vi "Read Init Motor Data.vi"(8 "error in (no error)":errorcluster, 11 "SGDV_Ctrl_Class in":refnum<class "SGDV Motor.lvclass">) -> (0 "error out":errorcluster, 1 "Init Motor Data":T1, 2 "Get Serial Data?":bool, 3 "SGDV_Ctrl_Class out":refnum<class "SGDV Motor.lvclass">)   [LabVIEW 2013, in "SGDV_Ctrl_v13_lib.lvlib" / "SGDV Motor.lvclass"]
uses:
  SGDV Motor.lvclass
  Controls and General VIs/Init Motor Data.ctl
  SGDV Motor.lvclass/SGDV Motor.ctl
  Controls and General VIs/Delta FPGA Refnum.ctl
  <vilib>/myRIO/Common/Instrument Driver Framework/myRIO v1.0/Encoder/typedefs/Encoder Signal Mode.ctl
  <vilib>/rvi/interface/common/niFpgaWaitOnOcc.vi
  <vilib>/myRIO/Instrument Drivers/Onboard IO/Encoder/vis/Open.vi
  <vilib>/myRIO/Common/Instrument Driver Framework/myRIO v1.0/Encoder/vis/myRIO v1.1 Open Encoder.vi
  <vilib>/myRIO/Common/Instrument Driver Framework/myRIO v1.0/Encoder/vis/myRIO v1.0 Close Encoder.vi
  <vilib>/myRIO/Common/Instrument Driver Framework/Utilities/vis/Validate Channels.vi
  <vilib>/myRIO/Common/Instrument Driver Framework/myRIO v1.0/Encoder/vis/myRIO v1.0 Reserve Encoder.vi
  <vilib>/myRIO/Common/Instrument Driver Framework/myRIO v1.0/Encoder/vis/myRIO v1.0 Unreserve Encoder.vi
  <vilib>/myRIO/Common/Instrument Driver Framework/myRIO v1.0/Encoder/vis/myRIO v1.0 Build MUX Configuration Encoder.vi
  <vilib>/myRIO/Common/Instrument Driver Framework/myRIO v1.0/Resource Manager/vis/myRIO v1.0 Reserve Channel List.vi
  <vilib>/myRIO/Common/Instrument Driver Framework/myRIO v1.0/Resource Manager/vis/myRIO v1.0 Unreserve Channel List.vi
  <vilib>/myRIO/Common/Instrument Driver Framework/myRIO v1.0/Resource Manager/vis/myRIO v1.0 Create Configuration List.vi
  <vilib>/myRIO/Common/Instrument Driver Framework/myRIO v1.0/Resource Manager/vis/myRIO v1.0 Reserve Channel.vi
  <vilib>/myRIO/Common/Instrument Driver Framework/myRIO v1.0/Resource Manager/vis/myRIO v1.0 Unreserve Channel.vi
  <vilib>/myRIO/Common/Instrument Driver Framework/myRIO v1.0/Resource Manager/vis/myRIO v1.0 Build Mutex Name.vi
  <vilib>/myRIO/Common/Instrument Driver Framework/myRIO v1.0/Encoder/vis/myRIO v1.0 Configure Encoder.vi
  <vilib>/myRIO/Common/Instrument Driver Framework/myRIO v1.0/myRIO v1.1 Open.vi
  <vilib>/Utility/VariantDataType/GetNumericInfo.vi
  <vilib>/Utility/error.llb/Error Cluster From Error Code.vi
  <vilib>/myRIO/Common/Instrument Driver Framework/Utilities/vis/IO Manager.vi
  <vilib>/myRIO/Common/Instrument Driver Framework/Utilities/vis/Configuration Manager.vi
  <vilib>/myRIO/Common/Instrument Driver Framework/myRIO v1.0/Resource Manager/vis/myRIO v1.0 Configure IO.vi
  <vilib>/myRIO/Common/Instrument Driver Framework/myRIO v1.0/myRIO v1.0 Close.vi
  <vilib>/myRIO/Common/Instrument Driver Framework/myRIO v1.0/Encoder/vis/myRIO v1.0 Shutdown Encoder.vi
  <vilib>/myRIO/Common/Instrument Driver Framework/myRIO v1.0/Encoder/vis/myRIO v1.0 Read Encoder.vi
  <vilib>/rvi/errors/niLvFpgaAdjustHostInterfaceError.vi
  <vilib>/rvi/interface/nirviReadWriteControl/nirviReadWriteControl.xnode
  <vilib>/rvi/interface/nirviMethod/nirviMethod.xnode
  SGDV_Ctrl_v13_lib.lvlib
  NiFpgaLv.dll
  <vilib>/rvi/interface/Simulation/niFpgaSimulationCallBeginRW.vi
  <vilib>/myRIO/Instrument Drivers/Onboard IO/Encoder/Encoder.lvlib
  <vilib>/FPGAPlugInAG/Dynamic/niLvFpga_ReadFifo_Dynamic.vi
  <vilib>/rvi/errors/niLvFpgaMergeErrorWithErrorCode.vi
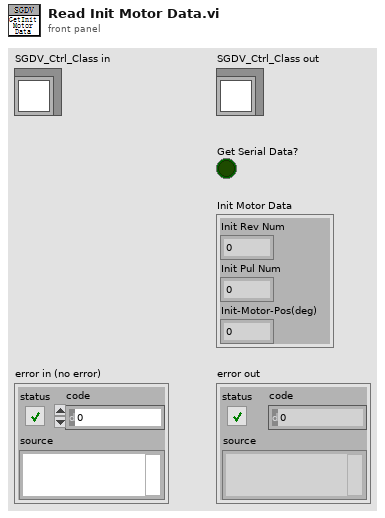
[diagram p1: front panel]
types:
  T1 = typedef "SGDV_Ctrl_v13_lib.lvlib/Init Motor Data.ctl" = cluster{"Init Rev Num":i32, "Init Pul Num":i32, "Init-Motor-Pos(deg)":dbl}
  T2 = typedef "Generic FPGA Reference.ctl" = refnum<k20>
  T3 = typedef "SGDV_Ctrl_v13_lib.lvlib/Delta FPGA Refnum.ctl" = refnum<k20>
  T4 = typedef "Encoder Signal Mode.ctl" = enum16{"Quadrature Phase Signal", "Step and Direction Signal"}
  T5 = typedef "Encoder.lvlib/Encoder Reference.ctl" = cluster{"myRIO Reference":T6, "Encoder Channels Enum":T9}
  T6 = typedef "myRIO Generic Hardware Reference.ctl" = cluster{"myRIO Model":T7, "myRIO Hardware Reference":T8}
  T7 = typedef "Hardware Version Enum.ctl" = enum16{"Unknown", "myRIO-1900", "myRIO-1950"}
  T8 = typedef "myRIO v1.0 Reference.ctl" = cluster{"Generic FPGA Reference":T2, "Allow multiple opens":bool}
  T9 = typedef "Encoder Channels Enum.ctl" = enum16{"Not Connected", "C/ENC0", "C/ENC1", "A/ENC", "B/ENC"}
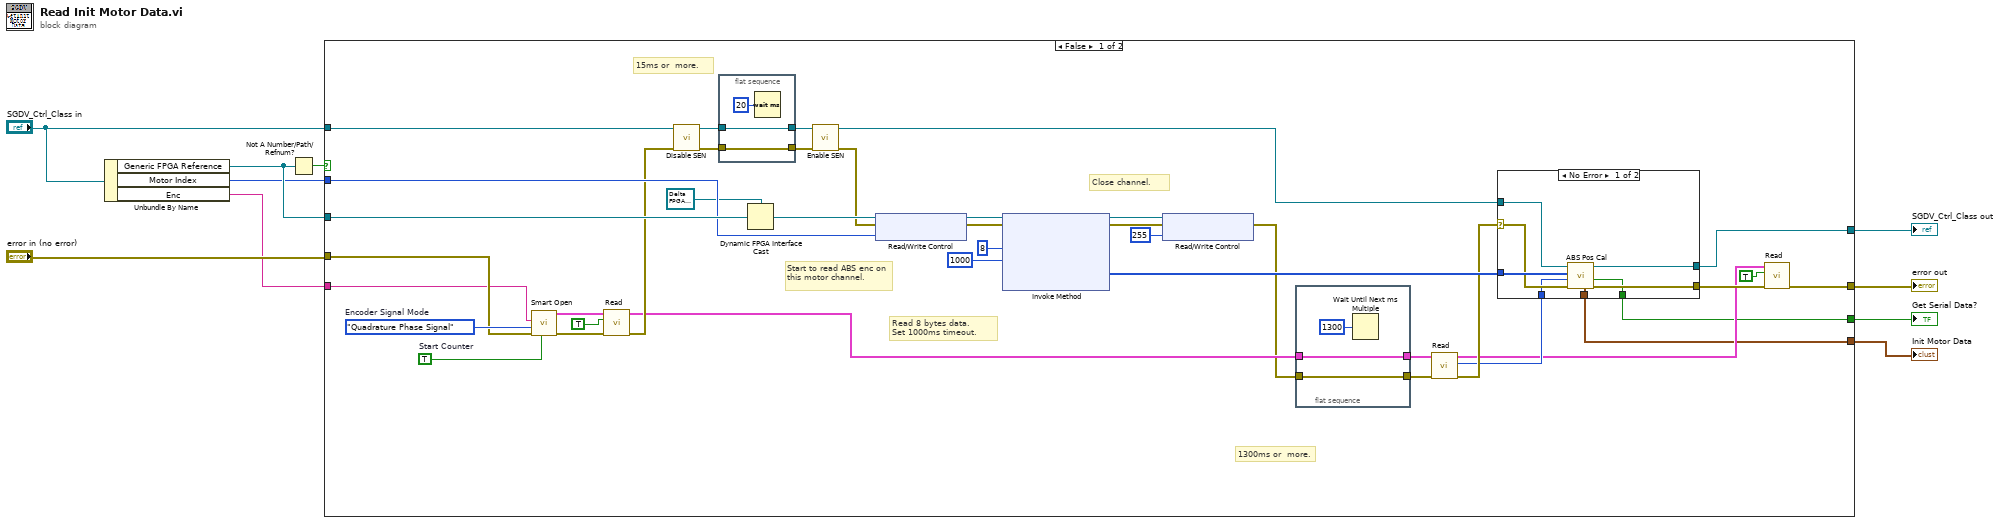
[diagram p0: block diagram]
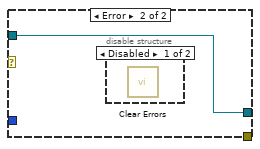
[diagram p2: hidden frame]
diagram:
  n1 = Unbundle By Name("SGDV_Ctrl_Class in") -> ("Generic FPGA Reference"=w9:T2, "Motor Index"=w8:u8, "Enc"=w1:tag)
  n2 = Not A Number/Path/Refnum?(number/path/refnum=w9) -> (NaN/Path/Refnum?=w10:bool)
  n3 = case shown="False" w10 {
    tunnel: w9 -> [w50 _]
    tunnel: "SGDV_Ctrl_Class in" -> [w21 w67]
    tunnel: "error in (no error)" -> [w18 w66]
    tunnel: w8 -> [w49 _]
    tunnel: [w23 w67] -> w4
    tunnel: [w27 w66] -> w7
    tunnel: [w24 _] -> w3
    tunnel: [w22 _] -> w2
    tunnel: w1 -> [w11 _]
    frame False {
      w33 = TRUE  # Start Counter
      w41 = Encoder_Signal_Mode."Quadrature Phase Signal"  # Encoder Signal Mode
      # "1300ms or  more."
      # "Close channel."
      # "15ms or  more."
      # "Read 8 bytes data.\nSet 1000ms timeout."
      # "Start to read ABS enc on this motor channel."
      n4 = call <vilib>:"Smart Open.vi"("Start Counter"=w33, "error in (no error)"=w18, "Encoder Signal Mode"=w41, "Channel Name"=w11) -> ("error out"=w16:errorcluster, "Encoder Ref Out"=w17:T5)  [unwired: 6 in]
      n5 = call <vilib>:"Read.vi"("error in (no error)"=w16, "Reset Counter"=TRUE, "Encoder Ref In"=w17) -> ("error out"=w15:errorcluster, "Encoder Ref Out"=w14:T5)  [unwired: 4 in, 3 out]
      n6 = call "Disable SEN.vi"("error in (no error)"=w15, "SGDV_Ctrl_Class in"=w21) -> ("error out"=w19:errorcluster, "SGDV_Ctrl_Class out"=w20:refnum<class "SGDV Motor.lvclass">)  [unwired: 8 in]
      n7 = flat-sequence {
        tunnel: w20 -> [w51]
        tunnel: w19 -> [w52]
        tunnel: [w52] -> w37
        tunnel: [w51] -> w38
        frame #0 {
          n8 = Wait (ms)(milliseconds to wait=u32 20) -> ()  [unwired: 1 out]
        }
      }
      n9 = Dynamic FPGA Interface Cast(Session In=T3 refnum ("Delta FPGA Refnum"), Type=w50) -> (Session Out=w43:T3)
      n10 = call "Enable SEN.vi"("error in (no error)"=w37, "SGDV_Ctrl_Class in"=w38) -> ("error out"=w42:errorcluster, "SGDV_Ctrl_Class out"=w32:refnum<class "SGDV Motor.lvclass">)  [unwired: 8 in]
      n11 = xnode "Read/Write Control"("FPGA VI Reference In"=w43, "error in"=w42, "ABS Enc Channel"=w49) -> ("FPGA VI Reference Out"=w48:T3, "error out"=w44:errorcluster)
      n12 = xnode "Invoke Method"("FPGA VI Reference In"=w48, "error in"=w44, "Number of Elements"=u32 8, "Timeout (ms)"=1000) -> ("FPGA VI Reference Out"=w45:T3, "error out"=w39:errorcluster, "Data"=w46:u8[])  [unwired: 1 out]
      n13 = xnode "Read/Write Control"("FPGA VI Reference In"=w45, "error in"=w39, "ABS Enc Channel"=u8 255) -> ("error out"=w13:errorcluster)  [unwired: 1 out]
      n14 = flat-sequence {
        tunnel: w13 -> [w55]
        tunnel: [w55] -> w40
        tunnel: w14 -> [w54]
        tunnel: [w54] -> w31
        frame #0 {
          n15 = Wait Until Next ms Multiple(millisecond multiple=u32 1300) -> ()  [unwired: 1 out]
        }
      }
      n16 = call <vilib>:"Read.vi"("error in (no error)"=w40, "Encoder Ref In"=w31) -> ("error out"=w30:errorcluster, "Counter Value"=w29:i32, "Encoder Ref Out"=w26:T5)  [unwired: 5 in, 2 out]
      n17 = case shown="No Error" w30 {
        selector: w30 -> [w63 _]
        tunnel: w46 -> [w64 _]
        tunnel: [w62 _] -> w28
        tunnel: w32 -> [w61 w65]
        tunnel: [w60 w65] -> w23
        tunnel: w29 -> [w59 _]
        tunnel: [w58 _] -> w24
        tunnel: [w57 _] -> w22
        frame No Error {
          n18 = call "ABS Pos Cal.vi"("error in (no error)"=w63, "Init Pul Num"=w59, "Data"=w64, "SGDV_Ctrl_Class in"=w61) -> ("error out"=w62:errorcluster, "Get Serial Data?"=w58:bool, "SGDV_Ctrl_Class out"=w60:refnum<class "SGDV Motor.lvclass">, "Init Motor Data"=w57:T1)  [unwired: 3 in, 1 out]
        }
        frame Error {
          n19 = disable-structure shown="Disabled" {
            frame Disabled {
              n20 = call <vilib>:"Clear Errors.vi"() -> ()  [unwired: 7 in, 1 out]
            }
            frame Enabled {
            }
          }
        }
      }
      n21 = call <vilib>:"Read.vi"("error in (no error)"=w28, "Reset Counter"=TRUE, "Encoder Ref In"=w26) -> ("error out"=w27:errorcluster)  [unwired: 4 in, 4 out]
    }
    frame True {
    }
  }
  "SGDV_Ctrl_Class out" <- w4
  "error out" <- w7
  "Get Serial Data?" <- w3
  "Init Motor Data" <- w2
